vi "Player Info.vi"(11 "Assassin in":refnum<class "Assassin.lvclass">) -> (0 "Defeat Speech":string, 1 "Victory Speech":string, 2 "Name":string, 3 "Assassin out":refnum<class "Assassin.lvclass">)   [LabVIEW 2015, in "Assassin.lvclass"]
uses:
  Assassin.lvclass
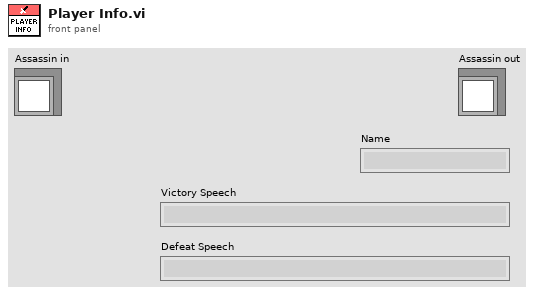
[diagram p1: front panel]
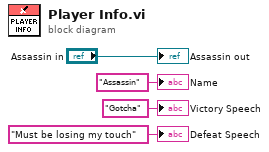
[diagram p0: block diagram]
diagram:
  "Assassin out" <- "Assassin in"
  "Name" <- "Assassin" ("Name")
  "Victory Speech" <- "Gotcha" ("Victory Speech")
  "Defeat Speech" <- "Must be losing my touch" ("Defeat Speech")
